vi "Interruption.vi"(8 "Duration":sgl, 10 "Position":dbl, 11 "Sine":sgl[](array[numeric])) -> (3 "Sine+Anomaly":sgl[](graph))   [LabVIEW 2020]
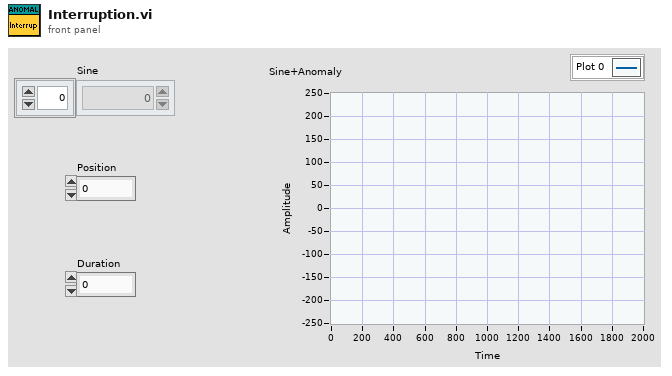
[diagram p1: front panel]
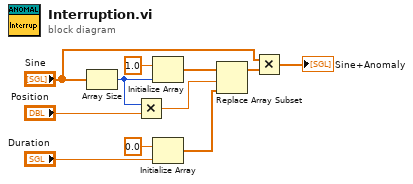
[diagram p0: block diagram]
diagram:
  n1 = Array Size(array="Sine") -> (size(s)=w5:i32)
  n2 = Multiply(x=w5, y="Position") -> (x*y=w1:dbl)
  n3 = Initialize Array(sgl 1.0 ("element"), w5) -> (w9:sgl[])
  n4 = Initialize Array(sgl 0.0 ("element"), "Duration") -> (w8:sgl[])
  n5 = Replace Array Subset(array=w9, new element=w8, index=w1) -> (w7:sgl[])
  n6 = Multiply(x="Sine", y=w7) -> (x*y=→"Sine+Anomaly":sgl[])
